vi "Create Loader.vi"(6 "timeout (ms)":i32=5000, 8 "error in":errorcluster, 10 "Loader Info":T1, 11 "gRPC ID in":T3) -> (0 "error out":errorcluster, 3 "gRPC ID out":T3)   [LabVIEW 2021, in "CIFManagerClientWrapper.lvlib"]
uses:
  CIFManagerClientWrapper.lvlib
  <vilib>/gRPC/LabVIEW gRPC Library/Shared/grpcId.ctl
  CIF_Manager_client/RPC Messages/cif_management_common_LoaderInfo.ctl
  CIF_Manager_client/RPC Messages/cif_management_common_LoaderType.ctl
  CIF_Manager_client/RPC Messages/cif_manager_CreatePluginLoaderRequest.ctl
  CIF_Manager_client/CIF_Manager_client.lvlib
  <vilib>/gRPC/LabVIEW gRPC Library/grpc-lvsupport-release.lvlib
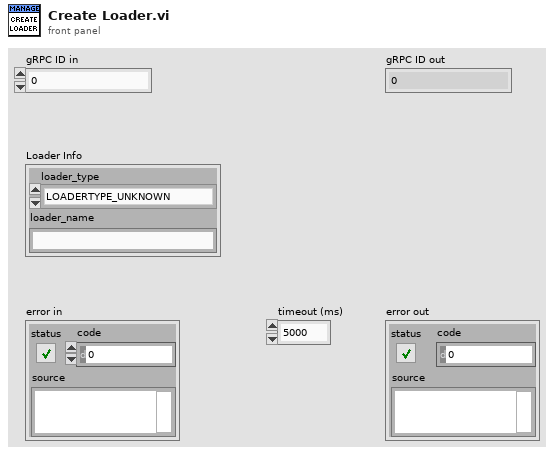
[diagram p1: front panel]
types:
  T1 = typedef "CIF_Manager_client.lvlib/cif_management_common_LoaderInfo.ctl" = cluster{"loader_type":T2, "loader_name":string}
  T2 = typedef "CIF_Manager_client.lvlib/cif_management_common_LoaderType.ctl" = enum32{"LOADERTYPE_UNKNOWN", "LOADERTYPE_LABVIEW"}
  T3 = typedef "grpc-lvsupport-release.lvlib/grpcId.ctl" = u64
  T4 = typedef "CIF_Manager_client.lvlib/cif_manager_CreatePluginLoaderRequest.ctl" = cluster{"loader_info":T1}
  T5 = typedef "CIF_Manager_client.lvlib/cif_manager_CreatePluginLoaderResponse.ctl" = cluster{"status":T6}
  T6 = typedef "CIF_Manager_client.lvlib/cif_common_Status.ctl" = cluster{"code":i32, "message":string}
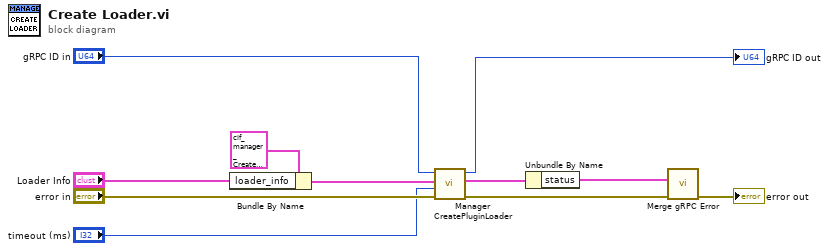
[diagram p0: block diagram]
diagram:
  n1 = Bundle By Name(cluster=T4 {"loader_info"={"loader_type"=enum."LOADERTYPE_UNKNOWN", "loader_name"=""}} ("Request Data"), "loader_info"="Loader Info") -> (w2:T4)
  n2 = call "Manager CreatePluginLoader.vi"("error in"="error in", "timeout (ms)"="timeout (ms)", "Request Data"=w2, "gRPC ID"="gRPC ID in") -> ("error out"=w7:errorcluster, "Response Data"=w5:T5, "gRPC ID out"=→"gRPC ID out":T3)  [unwired: 5 in]
  n3 = Unbundle By Name(w5) -> ("status"=w4:T6)
  n4 = call "Merge gRPC Error.vi"("error in (no error)"=w7, "gRPC Error"=w4) -> ("error out"=→"error out":errorcluster)  [unwired: 9 in]
